vi "c vs time graphing.vi"() -> (8 "C vs time graph":cluster{dbl[], dbl[]})   [LabVIEW 2019]
doc: "This is a Bug C(T) subVI.\n\nIt creates the capacitance versus the time graph.\n\nPaul K Dixon\nP3600\nCSUSB Physics"
uses:
  globals/Bug globals.vi
panel:
  # "needs \nwork\ninside"
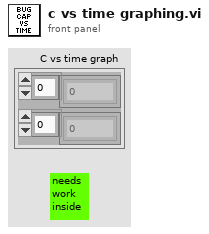
[diagram p1: front panel]
types:
  T1 = typedef "result.ctl" = cluster{"Temp (C)":dbl, "RC Fit":T2, "wave":waveform(dbl), "Time (s)":dbl}
  T2 = typedef "cap fit params.ctl" = cluster{"Resistance (Ohms)":dbl, "Est Time constant (s)":dbl, "Est Capacitance (F)":dbl}
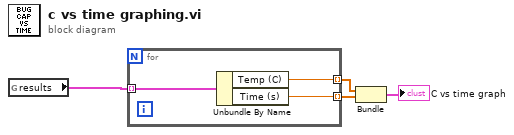
[diagram p0: block diagram]
diagram:
  n1 = global read "Bug globals.vi" "results"() -> (w4:T1[])
  n2 = for {
    tunnel: w4 -> [w7] mode=indexing
    tunnel: [w6] -> w3 mode=indexing
    tunnel: [w5] -> w2 mode=indexing
    n3 = Unbundle By Name(w7) -> ("Temp (C)"=w6:dbl, "Time (s)"=w5:dbl)
  }
  n4 = Bundle(w3, w2) -> (→"C vs time graph":cluster{dbl[], dbl[]})  [unwired: 1 in]
